vi "End.vi"(8 "error in (no error)":errorcluster, 11 "SPARC4_GUI in":refnum<class "SPARC4_GEI.lvclass">) -> (0 "error out":errorcluster, 3 "SPARC4_GUI out":refnum<class "SPARC4_GEI.lvclass">)   [LabVIEW 2018, in "SPARC4_GEI.lvclass"]
uses:
  SPARC4_GEI.lvclass
  SPARC4_GEI.lvclass/SPARC4_GEI.ctl
  Channel GUI/Channel GEI.lvclass
  Filter_Wheel/Filter_Wheel.lvclass
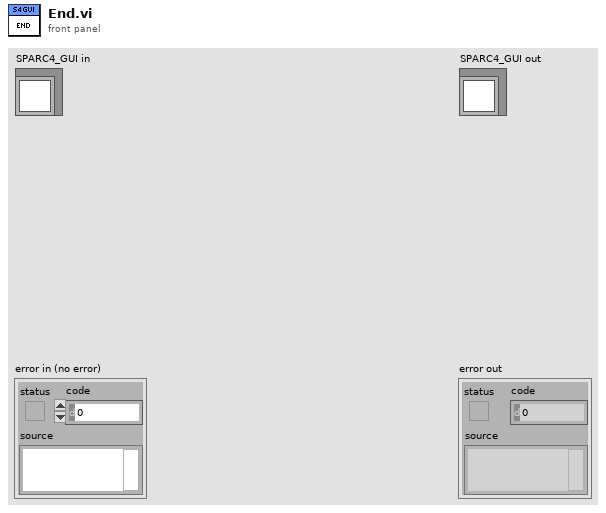
[diagram p1: front panel]
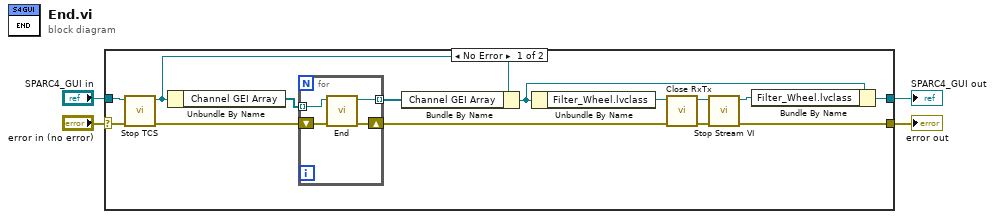
[diagram p0: block diagram]
diagram:
  n1 = case shown="No Error" "error in (no error)" {
    selector: "error in (no error)" -> [w15 w24]
    tunnel: [w7 w24] -> w3
    tunnel: [w11 w23] -> w1
    tunnel: "SPARC4_GUI in" -> [w16 w23]
    frame No Error {
      n2 = call "Stop TCS.vi"("error in (no error)"=w15, "SPARC4_GEI in"=w16) -> ("error out"=w14:errorcluster, "SPARC4_GEI out"=w13:refnum<class "SPARC4_GEI.lvclass">)  [unwired: 8 in]
      n3 = Unbundle By Name(w13) -> ("Channel GEI Array"=w17:refnum<class "Channel GEI.lvclass">[])
      n4 = for {
        tunnel: [w20] -> w18 mode=indexing
        tunnel: w17 -> [w19] mode=indexing
        shift-right: [w21] -> w5
        shift-left: w14 -> [w22]
        n5 = call "End.vi"("error in (no error)"=w22, "Channel GUI in"=w19) -> ("error out"=w21:errorcluster, "Channel GUI out"=w20:refnum<class "Channel GEI.lvclass">)  [unwired: 8 in]
      }
      n6 = Bundle By Name(cluster=w13, "Channel GEI Array"=w18) -> (w12:refnum<class "SPARC4_GEI.lvclass">)
      n7 = Unbundle By Name(w12) -> ("Filter_Wheel.lvclass"=w10:refnum<class "Filter_Wheel.lvclass">)
      n8 = call "Close RxTx.vi"("error in (no error)"=w5, "Filter_Wheel in"=w10) -> ("error out"=w6:errorcluster, "Filter_Wheel out"=w9:refnum<class "Filter_Wheel.lvclass">)  [unwired: 8 in]
      n9 = call "Stop Stream VI.vi"("error in (no error)"=w6, "Filter_Wheel in"=w9) -> ("error out"=w7:errorcluster, "Filter_Wheel out"=w8:refnum<class "Filter_Wheel.lvclass">)  [unwired: 8 in]
      n10 = Bundle By Name(cluster=w12, "Filter_Wheel.lvclass"=w8) -> (w11:refnum<class "SPARC4_GEI.lvclass">)
    }
    frame Error {
    }
  }
  "error out" <- w3
  "SPARC4_GUI out" <- w1
